vi "表换线提示.vi"(8 "error in (no error)":errorcluster caption="错误输入（无错误）", 9 "型号":string="接线图\\Simulation DMM", 10 "接线状态":i32, 11 "数字多用表接口 输入":refnum<class "数字多用表接口.lvclass">) -> (0 "error out":errorcluster caption="错误输出", 3 "数字多用表接口 输出":refnum<class "数字多用表接口.lvclass">)   [LabVIEW 2020, in "数字多用表接口.lvlib" / "数字多用表接口.lvclass"]
uses:
  <vilib>/Utility/miscctls.llb/LVBoundsTypeDef.ctl
  <vilib>/Utility/miscctls.llb/LVRectTypeDef.ctl
panel:
  in  "Path 2":path=path "D:/项目/2023项目/柳州长虹/数字多用表自动化程序/接线图/Simulation DMM/1.png"
  out "2D Picture":picture
  in  "Button":bool
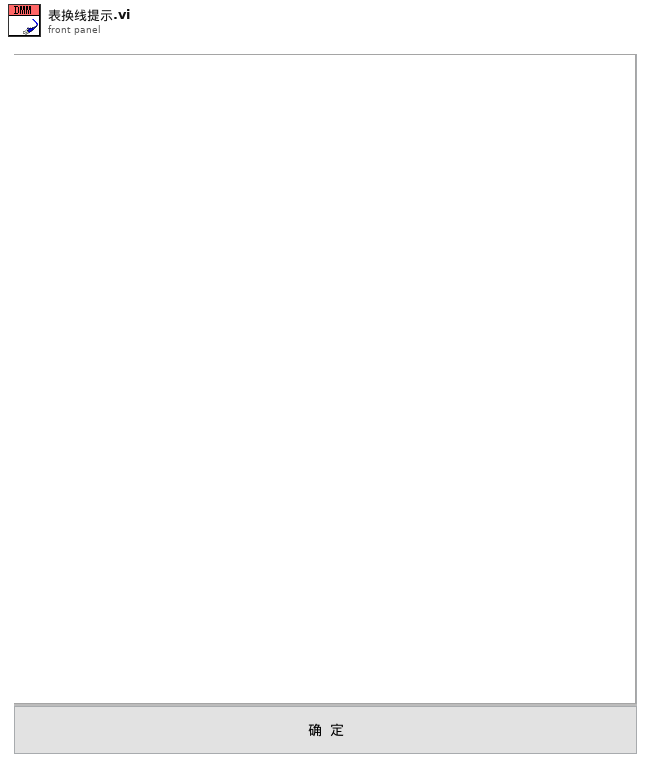
[diagram p1: front panel]
types:
  T1 = typedef "LVRectTypeDef.ctl" = cluster{"Left":i16, "Top":i16, "Right":i16, "Bottom":i16}
  T2 = typedef "LVBoundsTypeDef.ctl" = cluster{"Width":u32, "Height":u32}
  T3 = typedef "imagedata.ctl" = cluster{"image type":i32, "image depth":i32, "image":u8[], "mask":u8[], "colors":u32[], "Rectangle":cluster{"left":i16, "top":i16, "right":i16, "bottom":i16}}
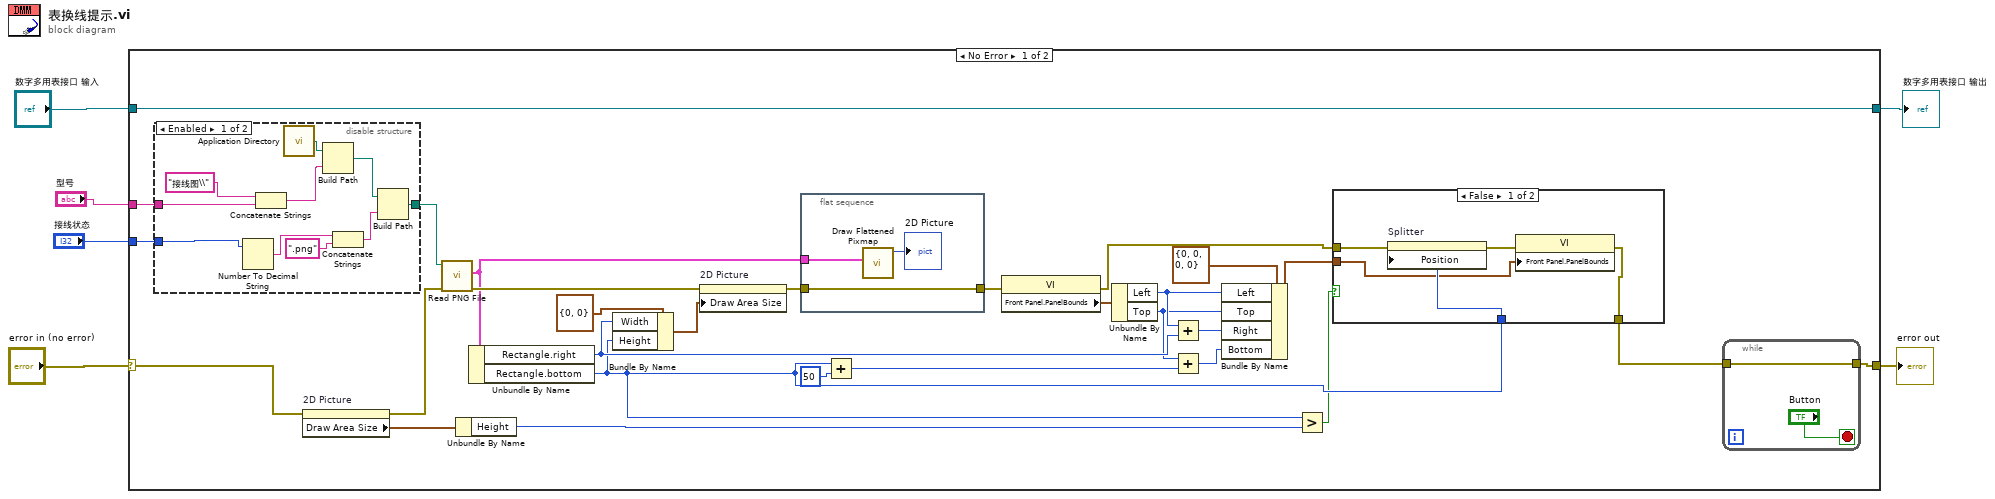
[diagram p0: block diagram]
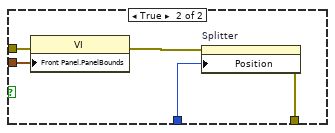
[diagram p2: hidden frame]
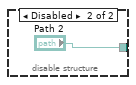
[diagram p3: hidden frame]
diagram:
  n1 = case shown="No Error" "error in (no error)" {
    selector: "error in (no error)" -> [w13 w63]
    tunnel: [w18 w63] -> w5
    tunnel: [w35 w62] -> w3
    tunnel: "数字多用表接口 输入" -> [w35 w62]
    tunnel: "接线状态" -> [w19 _]
    tunnel: "型号" -> [w17 _]
    frame No Error {
      n2 = disable-structure shown="Enabled" {
        disable-tunnel: [w53 "Path 2"] -> w20
        disable-tunnel: w19 -> [w52 _]
        disable-tunnel: w17 -> [w51 _]
        frame Enabled {
          n3 = Number To Decimal String(number=w52) -> (decimal integer string=w56:string)  [unwired: 1 in]
          n4 = Concatenate Strings("接线图\\", w51) -> (w49:string)
          n5 = call <vilib>:"Application Directory.vi"() -> ("Application Directory"=w58:path)
          n6 = Build Path(base path=w58, name or relative path=w49) -> (appended path=w57:path)
          n7 = Concatenate Strings(w56, ".png" ("string")) -> (w54:string)
          n8 = Build Path(base path=w57, name or relative path=w54) -> (appended path=w53:path)
        }
        frame Disabled {
        }
      }
      n9 = property on="2D Picture" class="Pict"(error in=w13) -> (error out=w12:errorcluster, "Draw Area Size"=w11:T2)  [unwired: 1 in, 1 out]
      n10 = call <vilib>:"Read PNG File.vi"("error in (no error)"=w12, "path to PNG file"=w20) -> ("error out"=w32:errorcluster, "image data"=w22:T3)  [unwired: 7 in, 1 out]
      n11 = Unbundle By Name(w11) -> ("Height"=w9:u32)
      n12 = Unbundle By Name(w22) -> ("Rectangle.right"=w28:i16, "Rectangle.bottom"=w10:i16)
      n13 = Bundle By Name(cluster=T2 {"Width"=0, "Height"=0} ("Draw Area Size"), "Width"=w28, "Height"=w10) -> (w15:T2)
      n14 = property on="2D Picture" class="Pict"(error in=w32, "Draw Area Size"=w15) -> (error out=w14:errorcluster)  [unwired: 1 in, 1 out]
      n15 = flat-sequence {
        tunnel: [w47] -> w21
        tunnel: w14 -> [w47]
        tunnel: w22 -> [w46]
        frame #0 {
          n16 = call <vilib>:"Draw Flattened Pixmap.vi"("image data"=w46) -> ("new picture"=→"2D Picture":picture)  [unwired: 8 in]
        }
      }
      n17 = Add(x=w10, y=i16 50 ("x")) -> (x+y=w25:i16)
      n18 = property class="VI"(error in=w21) -> (error out=w16:errorcluster, "Front Panel.PanelBounds"=w31:T1)  [unwired: 1 in, 1 out]
      n19 = Unbundle By Name(w31) -> ("Left"=w29:i16, "Top"=w26:i16)
      n20 = Add(x=w29, y=w28) -> (x+y=w27:i16)
      n21 = Add(x=w26, y=w25) -> (x+y=w24:i16)
      n22 = Bundle By Name(cluster=T1 {"Left"=0, "Top"=0, "Right"=0, "Bottom"=0} ("Front Panel Window:Panel Bounds"), "Left"=w29, "Top"=w26, "Right"=w27, "Bottom"=w24) -> (w23:T1)
      n23 = Greater?(x=w10, y=w9) -> (0:w7:bool)
      n24 = case shown="False" w7 {
        tunnel: w23 -> [w37 w45]
        tunnel: w16 -> [w39 w44]
        tunnel: w10 -> [w38 w42]
        tunnel: [w36 w41] -> w8
        frame False {
          n25 = property on="Splitter" class="Splitter"(error in=w39, "Position"=w38) -> (error out=w40:errorcluster)  [unwired: 1 in, 1 out]
          n26 = property class="VI"(error in=w40, "Front Panel.PanelBounds"=w37) -> (error out=w36:errorcluster)  [unwired: 1 in, 1 out]
        }
        frame True {
          n27 = property class="VI"(error in=w44, "Front Panel.PanelBounds"=w45) -> (error out=w43:errorcluster)  [unwired: 1 in, 1 out]
          n28 = property on="Splitter" class="Splitter"(error in=w43, "Position"=w42) -> (error out=w41:errorcluster)  [unwired: 1 in, 1 out]
        }
      }
      n29 = while {
        tunnel: w8 -> [w60]
        tunnel: [w60] -> w18
        stop <- "Button" stop-if-true
      }
    }
    frame Error {
    }
  }
  "error out" <- w5
  "数字多用表接口 输出" <- w3
